vi "FPGA Read Sonars.vi"() -> (0 "Read Ready":bool, 1 "Time of Flight Front":u32, 2 "Time of Flight Right":u32, 3 "Time of Flight Back":u32, 4 "Time of Flight Left":u32)   [LabVIEW 2015]
uses:
  <vilib>/rvi/Emulation/niFpgaGetClockAttributes.vi
  <vilib>/rvi/Emulation/niFpgaSctlEmulationGetInTimedLoop.vi
  <vilib>/rvi/Emulation/niFpgaEmulationReportErrorSimple.vi
  <vilib>/rvi/eio/common/nirviEmuTemplateMethod_errors.vi
  <vilib>/rvi/Emulation/niFpgaProcessEmulError.vi
  <vilib>/rvi/Emulation/niFpgaCriticalErrorInLSC.vi
  <vilib>/eio/EIONode/EIONode.xnode
panel:
  out "Front Read":bool
  out "Right Read":bool
  out "Back Read":bool
  out "Left Read":bool
  in  "stop":bool
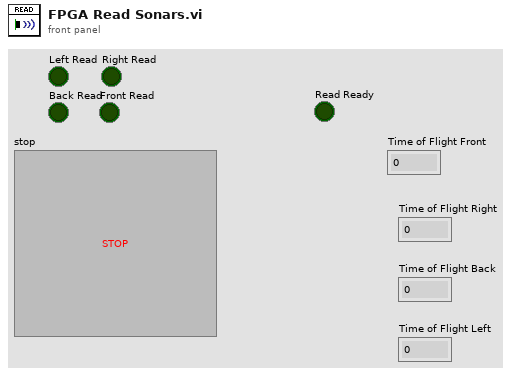
[diagram p1: front panel]
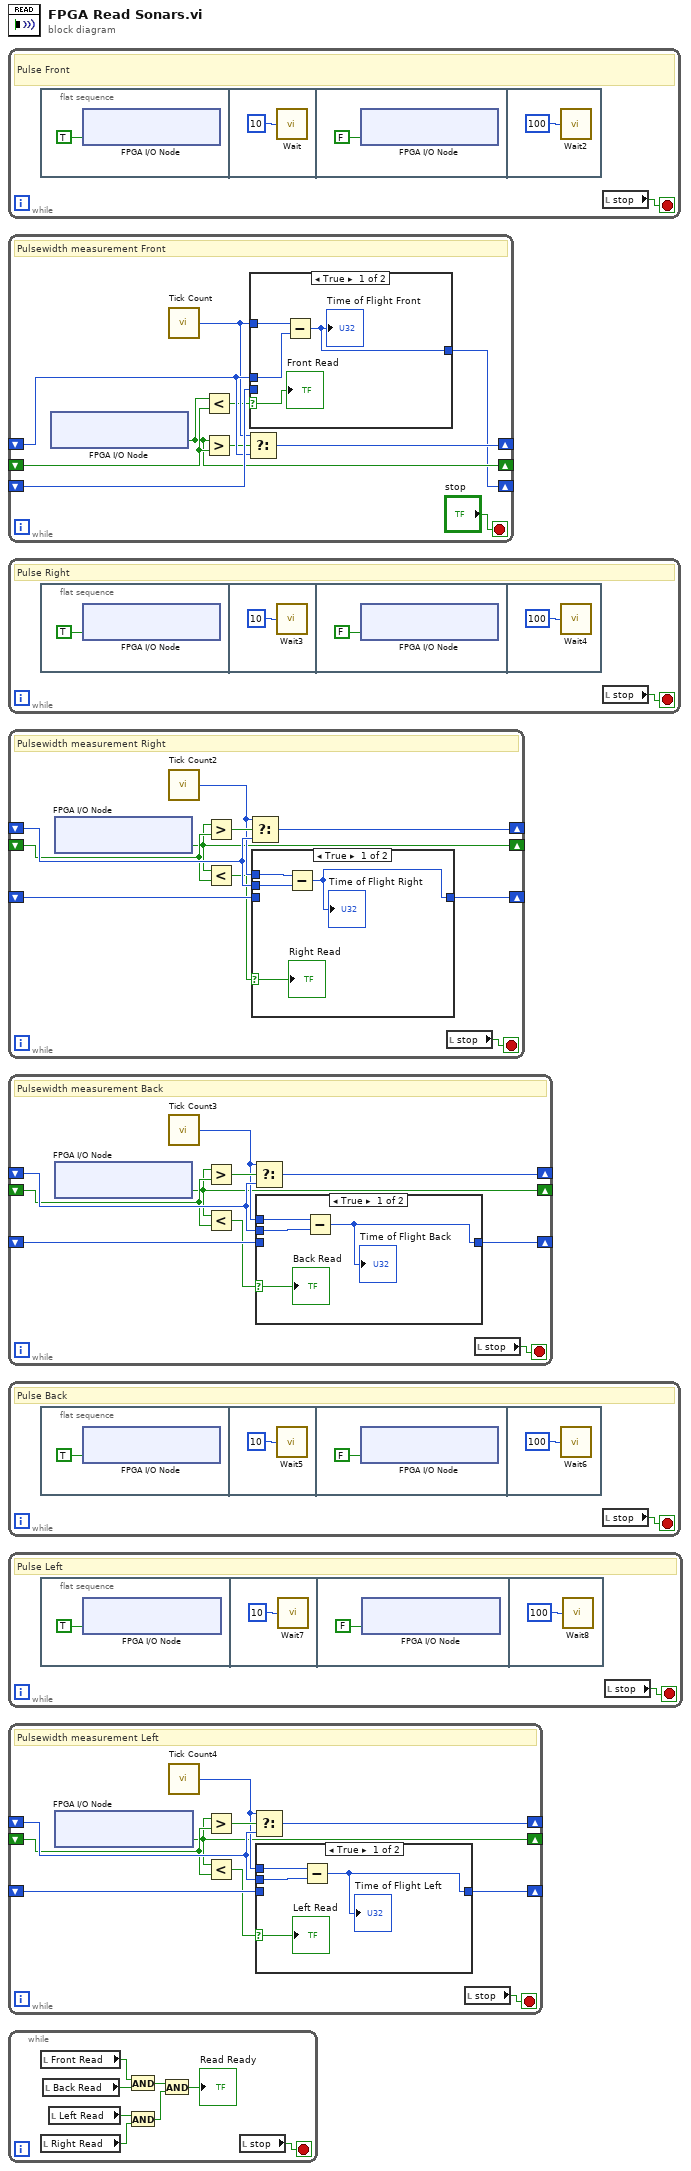
[diagram p0: block diagram]
diagram:
  n1 = while {
    stop <- w1 stop-if-true
    # "Pulse Front"
    n2 = flat-sequence {
      frame #0 {
        n3 = xnode "FPGA I/O Node"("ConnectorB/DIO4"=TRUE) -> ()  [unwired: 1 in, 1 out]
      }
      frame #1 {
        n4 = call "Wait"("Count(uSec)"=u32 10 ("Count(mSec)")) -> ()  [unwired: 1 out]
      }
      frame #2 {
        n5 = xnode "FPGA I/O Node"("ConnectorB/DIO4"=FALSE) -> ()  [unwired: 1 in, 1 out]
      }
      frame #3 {
        n6 = call "Wait2"("Count(mSec)"=u32 100) -> ()  [unwired: 1 out]
      }
    }
    n7 = local read "stop"() -> (w1:bool)
  }
  n8 = while "Pulsewidth Measurement + Sound Output" {
    shift-left: _ -> [w15]
    shift-right: [w7] -> _
    shift-left: _ -> [w14]
    shift-right: [w13] -> _
    shift-left: _ -> [w11]
    shift-right: [w8] -> _
    stop <- "stop" stop-if-true
    # "Pulsewidth measurement Front"
    n9 = xnode "FPGA I/O Node"() -> ("ConnectorB/DIO7"=w8:bool)  [unwired: 1 in, 1 out]
    n10 = call "Tick Count"() -> ("Tick Count(uSec)"=w10:u32)
    n11 = Less?(x=w8, y=w11) -> (x < y?=w9:bool)
    n12 = Greater?(x=w8, y=w11) -> (0:w12:bool)
    n13 = Select(t=w10, s=w12, f=w14) -> (s? t:f=w13:u32)
    n14 = case shown="True" w9 {
      selector: w9 -> [w16 _]
      tunnel: w15 -> [_ w20]
      tunnel: w10 -> [w18 _]
      tunnel: w14 -> [w19 _]
      tunnel: [w17 w20] -> w7
      frame True {
        n15 = Subtract(x=w18, y=w19) -> (x-y=w17:u32)
        "Time of Flight Front" <- w17
        "Front Read" <- w16
      }
      frame False {
      }
    }
  }
  n16 = while {
    stop <- w21 stop-if-true
    # "Pulse Right"
    n17 = flat-sequence {
      frame #0 {
        n18 = xnode "FPGA I/O Node"("ConnectorB/DIO3"=TRUE ("ConnectorB/DIO4")) -> ()  [unwired: 1 in, 1 out]
      }
      frame #1 {
        n19 = call "Wait3"("Count(uSec)"=u32 10 ("Count(mSec)")) -> ()  [unwired: 1 out]
      }
      frame #2 {
        n20 = xnode "FPGA I/O Node"("ConnectorB/DIO3"=FALSE ("ConnectorB/DIO4")) -> ()  [unwired: 1 in, 1 out]
      }
      frame #3 {
        n21 = call "Wait4"("Count(mSec)"=u32 100) -> ()  [unwired: 1 out]
      }
    }
    n22 = local read "stop"() -> (w21:bool)
  }
  n23 = while "Pulsewidth Measurement + Sound Output" {
    shift-left: _ -> [w35]
    shift-right: [w30] -> _
    shift-left: _ -> [w34]
    shift-right: [w33] -> _
    shift-left: _ -> [w31]
    shift-right: [w27] -> _
    stop <- w26 stop-if-true
    # "Pulsewidth measurement Right"
    n24 = xnode "FPGA I/O Node"() -> ("ConnectorB/DIO0"=w27:bool)  [unwired: 1 in, 1 out]
    n25 = call "Tick Count2"() -> ("Tick Count(uSec)"=w29:u32)
    n26 = Greater?(x=w27, y=w31) -> (0:w32:bool)
    n27 = Less?(x=w27, y=w31) -> (x < y?=w28:bool)
    n28 = Select(t=w29, s=w32, f=w34) -> (s? t:f=w33:u32)
    n29 = case shown="True" w28 {
      selector: w28 -> [w36 _]
      tunnel: w35 -> [_ w40]
      tunnel: w29 -> [w38 _]
      tunnel: w34 -> [w39 _]
      tunnel: [w37 w40] -> w30
      frame True {
        n30 = Subtract(x=w38, y=w39) -> (x-y=w37:u32)
        "Time of Flight Right" <- w37
        "Right Read" <- w36
      }
      frame False {
      }
    }
    n31 = local read "stop"() -> (w26:bool)
  }
  n32 = while "Pulsewidth Measurement + Sound Output" {
    shift-left: _ -> [w50]
    shift-right: [w45] -> _
    shift-left: _ -> [w49]
    shift-right: [w48] -> _
    shift-left: _ -> [w46]
    shift-right: [w42] -> _
    stop <- w41 stop-if-true
    # "Pulsewidth measurement Back"
    n33 = xnode "FPGA I/O Node"() -> ("ConnectorB/DIO1"=w42:bool)  [unwired: 1 in, 1 out]
    n34 = call "Tick Count3"() -> ("Tick Count(uSec)"=w44:u32)
    n35 = Greater?(x=w42, y=w46) -> (0:w47:bool)
    n36 = Less?(x=w42, y=w46) -> (x < y?=w43:bool)
    n37 = Select(t=w44, s=w47, f=w49) -> (s? t:f=w48:u32)
    n38 = case shown="True" w43 {
      selector: w43 -> [w51 _]
      tunnel: w50 -> [_ w55]
      tunnel: w44 -> [w53 _]
      tunnel: w49 -> [w54 _]
      tunnel: [w52 w55] -> w45
      frame True {
        n39 = Subtract(x=w53, y=w54) -> (x-y=w52:u32)
        "Time of Flight Back" <- w52
        "Back Read" <- w51
      }
      frame False {
      }
    }
    n40 = local read "stop"() -> (w41:bool)
  }
  n41 = while {
    stop <- w56 stop-if-true
    # "Pulse Back"
    n42 = flat-sequence {
      frame #0 {
        n43 = xnode "FPGA I/O Node"("ConnectorB/DIO2"=TRUE ("ConnectorB/DIO4")) -> ()  [unwired: 1 in, 1 out]
      }
      frame #1 {
        n44 = call "Wait5"("Count(uSec)"=u32 10 ("Count(mSec)")) -> ()  [unwired: 1 out]
      }
      frame #2 {
        n45 = xnode "FPGA I/O Node"("ConnectorB/DIO2"=FALSE ("ConnectorB/DIO4")) -> ()  [unwired: 1 in, 1 out]
      }
      frame #3 {
        n46 = call "Wait6"("Count(mSec)"=u32 100) -> ()  [unwired: 1 out]
      }
    }
    n47 = local read "stop"() -> (w56:bool)
  }
  n48 = while {
    stop <- w61 stop-if-true
    # "Pulse Left"
    n49 = flat-sequence {
      frame #0 {
        n50 = xnode "FPGA I/O Node"("ConnectorC/DIO1"=TRUE ("ConnectorB/DIO4")) -> ()  [unwired: 1 in, 1 out]
      }
      frame #1 {
        n51 = call "Wait7"("Count(uSec)"=u32 10 ("Count(mSec)")) -> ()  [unwired: 1 out]
      }
      frame #2 {
        n52 = xnode "FPGA I/O Node"("ConnectorC/DIO1"=FALSE ("ConnectorB/DIO4")) -> ()  [unwired: 1 in, 1 out]
      }
      frame #3 {
        n53 = call "Wait8"("Count(mSec)"=u32 100) -> ()  [unwired: 1 out]
      }
    }
    n54 = local read "stop"() -> (w61:bool)
  }
  n55 = while "Pulsewidth Measurement + Sound Output" {
    shift-left: _ -> [w75]
    shift-right: [w67] -> _
    shift-left: _ -> [w74]
    shift-right: [w73] -> _
    shift-left: _ -> [w71]
    shift-right: [w68] -> _
    stop <- w66 stop-if-true
    # "Pulsewidth measurement Left"
    n56 = xnode "FPGA I/O Node"() -> ("ConnectorC/DIO0"=w68:bool)  [unwired: 1 in, 1 out]
    n57 = call "Tick Count4"() -> ("Tick Count(uSec)"=w70:u32)
    n58 = Greater?(x=w68, y=w71) -> (0:w72:bool)
    n59 = Less?(x=w68, y=w71) -> (x < y?=w69:bool)
    n60 = Select(t=w70, s=w72, f=w74) -> (s? t:f=w73:u32)
    n61 = case shown="True" w69 {
      selector: w69 -> [w76 _]
      tunnel: w75 -> [_ w80]
      tunnel: w70 -> [w78 _]
      tunnel: w74 -> [w79 _]
      tunnel: [w77 w80] -> w67
      frame True {
        n62 = Subtract(x=w78, y=w79) -> (x-y=w77:u32)
        "Time of Flight Left" <- w77
        "Left Read" <- w76
      }
      frame False {
      }
    }
    n63 = local read "stop"() -> (w66:bool)
  }
  n64 = while {
    stop <- w81 stop-if-true
    n65 = local read "Front Read"() -> (w86:bool)
    n66 = local read "Right Read"() -> (w83:bool)
    n67 = local read "Back Read"() -> (w85:bool)
    n68 = local read "Left Read"() -> (w84:bool)
    n69 = And(x=w86, y=w85) -> (x .and. y?=w88:bool)
    n70 = And(x=w84, y=w83) -> (x .and. y?=w87:bool)
    n71 = And(x=w88, y=w87) -> (x .and. y?=→"Read Ready":bool)
    n72 = local read "stop"() -> (w81:bool)
  }
